vi "Check MongoDB Write --Unit Test.vi"(0 "Python Session":refnum<k35>, 5 "Python script path":path, 7 "Collection name":string, 9 "Expected JSON string":string, 11 "error in":errorcluster) -> (4 "Unit Test Result":cluster{"Message":string, "Passed?":bool}, 15 "error out":errorcluster)   [LabVIEW 2021]
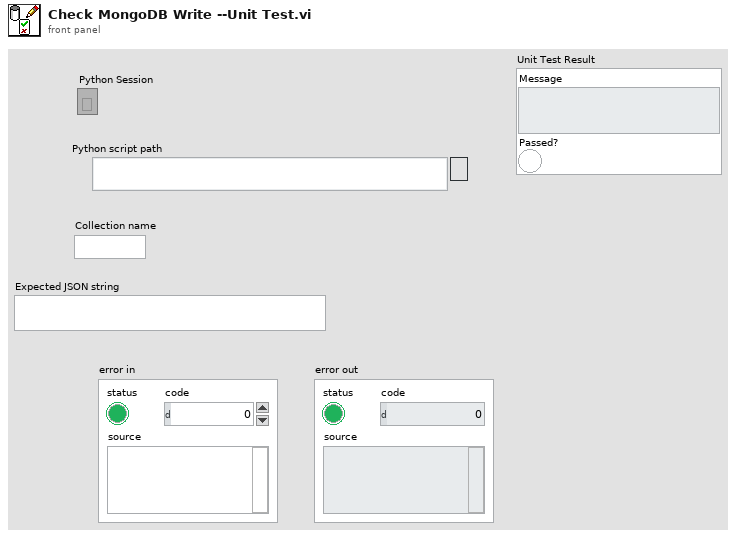
[diagram p1: front panel]
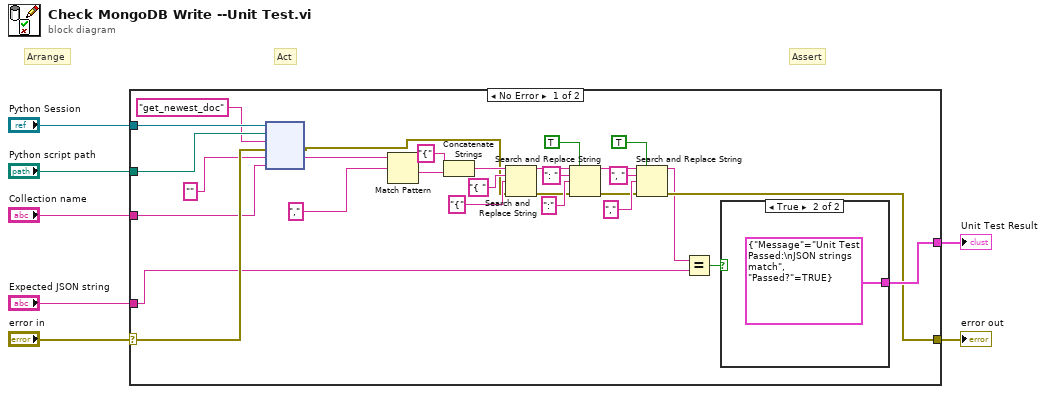
[diagram p0: block diagram]
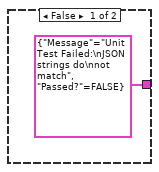
[diagram p2: hidden frame]
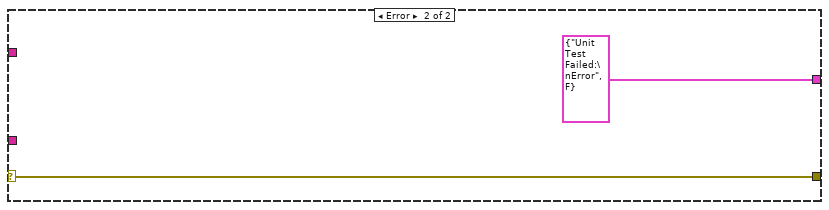
[diagram p3: hidden frame]
diagram:
  # "Assert"
  # "Act"
  # "Arrange"
  n1 = case shown="No Error" "error in" {
    selector: "error in" -> [w34 w40]
    tunnel: [w9 w40] -> w6
    tunnel: "Python Session" -> [w36 _]
    tunnel: "Python script path" -> [w35 _]
    tunnel: "Collection name" -> [w33 _]
    tunnel: "Expected JSON string" -> [w31 _]
    tunnel: [w29 cluster{"Message":string, "Passed?":bool} {"Message"="Unit Test Failed:\nError", "Passed?"=FALSE}] -> w1
    frame No Error {
      n2 = node(w36, w35, "get_newest_doc" ("function name"), w34, "", w33) -> (w12:errorcluster, w27:string)  [unwired: 1 in, 3 out]
      n3 = Match Pattern(string=w27, regular expression=",") -> (after substring=w24:string)  [unwired: 1 in, 3 out]
      n4 = Concatenate Strings("{" ("string"), w24) -> (w23:string)
      n5 = Search and Replace String(input string=w23, search string="{ ", replace string="{" ("replace string (\"\")"), error in=w12) -> (result string=w20:string, error out=w11:errorcluster)  [unwired: 4 in, 2 out]
      n6 = Search and Replace String(replace all?=TRUE ("replace all? (F)"), input string=w20, search string=": ", replace string=":" ("replace string (\"\")"), error in=w11) -> (result string=w16:string, error out=w10:errorcluster)  [unwired: 3 in, 2 out]
      n7 = Search and Replace String(replace all?=TRUE ("replace all? (F)"), input string=w16, search string=", ", replace string="," ("replace string (\"\")"), error in=w10) -> (result string=w8:string, error out=w9:errorcluster)  [unwired: 3 in, 2 out]
      n8 = Equal?(x=w8, y=w31) -> (x = y?=w30:bool)
      n9 = case shown="True" w30 {
        tunnel: [cluster{"Message":string, "Passed?":bool} {"Message"="Unit Test Failed:\nJSON strings do\nnot match", "Passed?"=FALSE} cluster{"Message":string, "Passed?":bool} {"Message"="Unit Test Passed:\nJSON strings match", "Passed?"=TRUE}] -> w29
        frame False {
        }
        frame True {
        }
      }
    }
    frame Error {
    }
  }
  "error out" <- w6
  "Unit Test Result" <- w1
